vi "Get Encoder Info.vi"(8 "error in (no error)":errorcluster, 11 "CIPC Reference":u64) -> (0 "error out":errorcluster, 3 "Encoder Info":T1)   [LabVIEW 2021, in "CIF_NI_CIPC.lvlib"]
uses:
  CIF_NI_CIPC.lvlib
  TypeDefs/Encoder Info.ctl
  libnicipc.dll
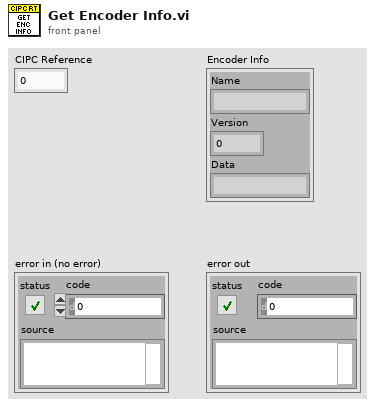
[diagram p1: front panel]
types:
  T1 = typedef "CIF_NI_CIPC.lvlib/Encoder Info.ctl" = cluster{"Name":string, "Version":i32, "Data":string}
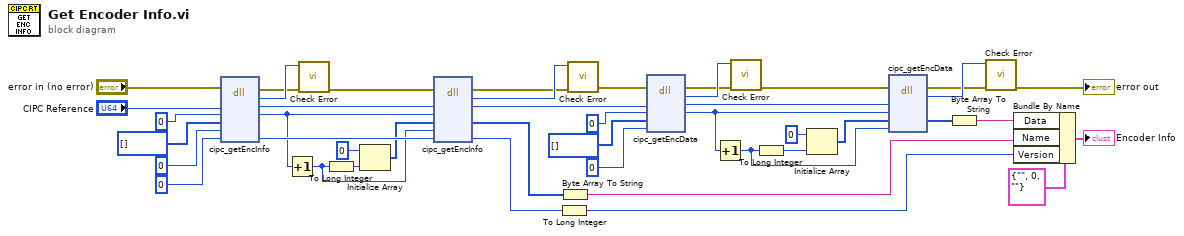
[diagram p0: block diagram]
diagram:
  n1 = dll-call lib="libnicipc.*" fn="cipc_getEncInfo"(error in="error in (no error)", "cipc_buffer_ref"="CIPC Reference", "enc_name_size"=u32 0 ("descr_size"), "enc_name"=u8[] [] ("initialized array"), "enc_name_maxsize"=u32 0 ("el_descr_maxsize"), "enc_version"=u32 0 ("head")) -> (error out=w42:errorcluster, "return type"=w43:i32, "cipc_buffer_ref"=w38:u64, "enc_name_size"=w34:u32, "enc_version"=w35:u32)  [unwired: 4 in, 1 out]
  n2 = Increment(x=w34) -> (x+1=w33:u32)
  n3 = call "Check Error.vi"("error in (no error)"=w42, "Error Code"=w43) -> ("error out"=w39:errorcluster)  [unwired: 9 in]
  n4 = To Long Integer(number=w33) -> (32bit integer=w7:i32)
  n5 = Initialize Array(u8 0, w7) -> (w31:u8[])
  n6 = dll-call lib="libnicipc.*" fn="cipc_getEncInfo"(error in=w39, "cipc_buffer_ref"=w38, "enc_name_size"=w34, "enc_name"=w31, "enc_name_maxsize"=w33, "enc_version"=w35) -> (error out=w40:errorcluster, "return type"=w41:i32, "cipc_buffer_ref"=w9:u64, "enc_name"=w30:u8[], "enc_version"=w32:u32)  [unwired: 4 in, 1 out]
  n7 = To Long Integer(number=w32) -> (32bit integer=w3:i32)
  n8 = Byte Array To String(unsigned byte array=w30) -> (string=w4:string)
  n9 = call "Check Error.vi"("error in (no error)"=w40, "Error Code"=w41) -> ("error out"=w8:errorcluster)  [unwired: 9 in]
  n10 = dll-call lib="libnicipc.*" fn="cipc_getEncData"(error in=w8, "cipc_buffer_ref"=w9, "enc_data_size"=u32 0 ("descr_size"), "enc_data"=u8[] [] ("initialized array"), "enc_data_maxsize"=u32 0 ("el_descr_maxsize")) -> (error out=w23:errorcluster, "return type"=w24:i32, "cipc_buffer_ref"=w19:u64, "enc_data_size"=w15:u32)  [unwired: 4 in, 1 out]
  n11 = Increment(x=w15) -> (x+1=w14:u32)
  n12 = call "Check Error.vi"("error in (no error)"=w23, "Error Code"=w24) -> ("error out"=w20:errorcluster)  [unwired: 9 in]
  n13 = To Long Integer(number=w14) -> (32bit integer=w6:i32)
  n14 = Initialize Array(u8 0, w6) -> (w13:u8[])
  n15 = dll-call lib="libnicipc.*" fn="cipc_getEncData"(error in=w20, "cipc_buffer_ref"=w19, "enc_data_size"=w15, "enc_data"=w13, "enc_data_maxsize"=w14) -> (error out=w21:errorcluster, "return type"=w22:i32, "enc_data"=w12:u8[])  [unwired: 5 in, 1 out]
  n16 = Byte Array To String(unsigned byte array=w12) -> (string=w10:string)
  n17 = call "Check Error.vi"("error in (no error)"=w21, "Error Code"=w22) -> ("error out"=→"error out":errorcluster)  [unwired: 9 in]
  n18 = Bundle By Name(cluster=T1 {"Name"="", "Version"=0, "Data"=""} ("Encoder Info 2"), "Data"=w10, "Name"=w4, "Version"=w3) -> (→"Encoder Info":T1)
